vi "Relays.vi"() -> ()   [LabVIEW 2011]
uses:
  low_level_proc/relaySpec.ctl
panel:
  out "As Gas":T2={"Remote"={"Card Index"=2, "Relay Index"=5}, "Active"={"Card Index"=2, "Relay Index"=6}, "Gas In"={"Card Index"=2, "Relay Index"=7}, "H2 Flush"={"Card Index"=2, "Relay Index"=8}, "Run"={"Card Index"=2, "Relay Index"=9}} {"Run"."Card Index" items=["1", "2", "3", "4", "5"]; "Run"."Relay Index" items=["1", "2", "3", "4", "5", "6", "7", "8", "9", "10", "11", "12"]; "H2 Flush"."Card Index" items=["1", "2", "3", "4", "5"]; "H2 Flush"."Relay Index" items=["1", "2", "3", "4", "5", "6", "7", "8", "9", "10", "11", "12"]; "Gas In"."Card Index" items=["1", "2", "3", "4", "5"]; "Gas In"."Relay Index" items=["1", "2", "3", "4", "5", "6", "7", "8", "9", "10", "11", "12"]; "Active"."Card Index" items=["1", "2", "3", "4", "5"]; "Active"."Relay Index" items=["1", "2", "3", "4", "5", "6", "7", "8", "9", "10", "11", "12"]; "Remote"."Card Index" items=["1", "2", "3", "4", "5"]; "Remote"."Relay Index" items=["1", "2", "3", "4", "5", "6", "7", "8", "9", "10", "11", "12"]}
  out "Al bubbler":T3={"Remote"={"Card Index"=0, "Relay Index"=3}, "Active"={"Card Index"=0, "Relay Index"=4}, "Bubbler In"={"Card Index"=0, "Relay Index"=5}, "Run"={"Card Index"=0, "Relay Index"=6}} {"Run"."Card Index" items=["1", "2", "3", "4", "5"]; "Run"."Relay Index" items=["1", "2", "3", "4", "5", "6", "7", "8", "9", "10", "11", "12"]; "Bubbler In"."Card Index" items=["1", "2", "3", "4", "5"]; "Bubbler In"."Relay Index" items=["1", "2", "3", "4", "5", "6", "7", "8", "9", "10", "11", "12"]; "Active"."Card Index" items=["1", "2", "3", "4", "5"]; "Active"."Relay Index" items=["1", "2", "3", "4", "5", "6", "7", "8", "9", "10", "11", "12"]; "Remote"."Card Index" items=["1", "2", "3", "4", "5"]; "Remote"."Relay Index" items=["1", "2", "3", "4", "5", "6", "7", "8", "9", "10", "11", "12"]}
  out "In bubbler":T3={"Remote"={"Card Index"=0, "Relay Index"=7}, "Active"={"Card Index"=0, "Relay Index"=8}, "Bubbler In"={"Card Index"=0, "Relay Index"=9}, "Run"={"Card Index"=0, "Relay Index"=10}} {"Run"."Card Index" items=["1", "2", "3", "4", "5"]; "Run"."Relay Index" items=["1", "2", "3", "4", "5", "6", "7", "8", "9", "10", "11", "12"]; "Bubbler In"."Card Index" items=["1", "2", "3", "4", "5"]; "Bubbler In"."Relay Index" items=["1", "2", "3", "4", "5", "6", "7", "8", "9", "10", "11", "12"]; "Active"."Card Index" items=["1", "2", "3", "4", "5"]; "Active"."Relay Index" items=["1", "2", "3", "4", "5", "6", "7", "8", "9", "10", "11", "12"]; "Remote"."Card Index" items=["1", "2", "3", "4", "5"]; "Remote"."Relay Index" items=["1", "2", "3", "4", "5", "6", "7", "8", "9", "10", "11", "12"]}
  out "Ga bubbler":T4={"Remote"={"Card Index"=3, "Relay Index"=0}, "Active"={"Card Index"=3, "Relay Index"=1}, "Bubbler In"={"Card Index"=3, "Relay Index"=2}, "Run"={"Card Index"=3, "Relay Index"=3}, "H2 Dilute"={"Card Index"=3, "Relay Index"=4}} {"H2 Dilute"."Card Index" items=["1", "2", "3", "4", "5"]; "H2 Dilute"."Relay Index" items=["1", "2", "3", "4", "5", "6", "7", "8", "9", "10", "11", "12"]; "Run"."Card Index" items=["1", "2", "3", "4", "5"]; "Run"."Relay Index" items=["1", "2", "3", "4", "5", "6", "7", "8", "9", "10", "11", "12"]; "Bubbler In"."Card Index" items=["1", "2", "3", "4", "5"]; "Bubbler In"."Relay Index" items=["1", "2", "3", "4", "5", "6", "7", "8", "9", "10", "11", "12"]; "Active"."Card Index" items=["1", "2", "3", "4", "5"]; "Active"."Relay Index" items=["1", "2", "3", "4", "5", "6", "7", "8", "9", "10", "11", "12"]; "Remote"."Card Index" items=["1", "2", "3", "4", "5"]; "Remote"."Relay Index" items=["1", "2", "3", "4", "5", "6", "7", "8", "9", "10", "11", "12"]}
  out "P Gas":T2={"Remote"={"Card Index"=2, "Relay Index"=0}, "Active"={"Card Index"=2, "Relay Index"=1}, "Gas In"={"Card Index"=2, "Relay Index"=2}, "H2 Flush"={"Card Index"=2, "Relay Index"=3}, "Run"={"Card Index"=2, "Relay Index"=4}} {"Run"."Card Index" items=["1", "2", "3", "4", "5"]; "Run"."Relay Index" items=["1", "2", "3", "4", "5", "6", "7", "8", "9", "10", "11", "12"]; "H2 Flush"."Card Index" items=["1", "2", "3", "4", "5"]; "H2 Flush"."Relay Index" items=["1", "2", "3", "4", "5", "6", "7", "8", "9", "10", "11", "12"]; "Gas In"."Card Index" items=["1", "2", "3", "4", "5"]; "Gas In"."Relay Index" items=["1", "2", "3", "4", "5", "6", "7", "8", "9", "10", "11", "12"]; "Active"."Card Index" items=["1", "2", "3", "4", "5"]; "Active"."Relay Index" items=["1", "2", "3", "4", "5", "6", "7", "8", "9", "10", "11", "12"]; "Remote"."Card Index" items=["1", "2", "3", "4", "5"]; "Remote"."Relay Index" items=["1", "2", "3", "4", "5", "6", "7", "8", "9", "10", "11", "12"]}
  # "Relay Card #"
  # "Relay Card #"
  # "Relay #"
  # "Relay #"
  # "Relay Card #"
  # "Relay #"
  # "Relay #"
  # "Relay Card #"
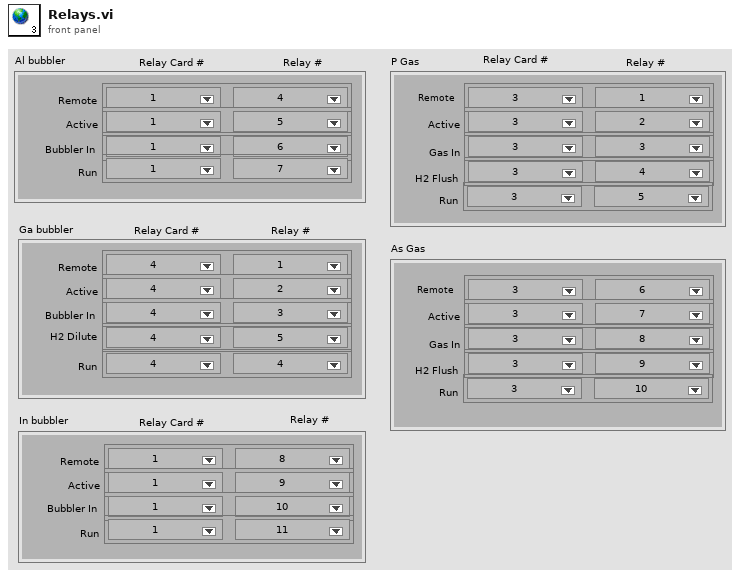
[diagram p1: front panel]
types:
  T1 = typedef "relaySpec.ctl" = cluster{"Card Index":u16, "Relay Index":u16}
  T2 = cluster{"Remote":T1, "Active":T1, "Gas In":T1, "H2 Flush":T1, "Run":T1}
  T3 = cluster{"Remote":T1, "Active":T1, "Bubbler In":T1, "Run":T1}
  T4 = cluster{"Remote":T1, "Active":T1, "Bubbler In":T1, "Run":T1, "H2 Dilute":T1}
diagram:
